vi "View AI param short.vi"(7 "ActivateAIView":bool, 9 "AIP":T1, 10 "AI_State":T3[](array[typedef]), 11 "AITable":dbl[](array[numeric]) format="%#.0f") -> (2 "Reread out":bool, 3 "This VI":refnum<vi>)   [LabVIEW 2019, in "Inputs.lvlib"]
uses:
  Inputs.lvlib
  Ctl/Parameter State.ctl
  Ctl/AI.ctl
  Ctl/AI short.ctl
  Database/Progress.vi
  Database/PostgreSQL.lvlib
  Logik/Logik.lvlib
panel:
  out "AI progress":i32(slide) scale=0.0..100.0
  in  "Reread":bool
  in  "n_elem":i32(c297)
  out "units":string[](array[string])
  out "AI_9":dbl format="%#.1f"
  out "AI_10":dbl format="%#.1f"
  out "AI_5":dbl format="%#.1f"
  out "AI_6":dbl format="%#.1f"
  out "AI_7":dbl format="%#.1f"
  out "AI_8":dbl format="%#.1f"
  out "AI_3":dbl format="%#.1f"
  out "AI_4":dbl format="%#.1f"
  out "AI_2":dbl format="%#.1f"
  out "AI_1":dbl format="%#.1f"
  out "n param":i32
  out "Names":string[](array[string])
  out "fcode":string[](array[string])
  out "Parameters table":dbl[][](array[numeric])=[[1.0, 0.0, 1000.0, 2.0, 0.0, 0.0, 2.0, 20.0, 100.0, nan, 250.0, 250.0, 2.0, 1.0, 10.0, 0.0, 65535.0, 0.0, 250.0, 1.0, 4.0], [1.0, 0.0, 1000.0, 2.0, 0.0, 0.0, 2.0, 20.0, 150.0, nan, 250.0, 250.0, 2.0, 1.0, 11.0, 0.0, 65535.0, 0.0, 250.0, 0.0, 4.0], [1.0, 0.0, 1000.0, 2.0, 0.0, 0.0, 2.0, 3.0, 7.0, 8.0, 10.0, 10.0, 2.0, 0.1, 1.0, 0.0, 65535.0, 0.0, 10.0, 0.0, 2.0], [1.0, 0.0, 1000.0, 2.0, 0.0, 0.0, 1.5, 2.5, 6.0, 7.0, 10.0, 10.0, 2.0, 0.1, 2.0, 0.0, 65535.0, 0.0, 10.0, 0.0, 3.0], [1.0, 0.0, 1000.0, 2.0, 0.0, 0.0, 2.0, 2.5, 6.0, 7.0, 10.0, 10.0, 2.0, 0.1, 3.0, 0.0, 65535.0, 0.0, 10.0, 1.0, 2.0], [1.0, 0.0, 1000.0, 2.0, 0.0, 0.0, 1.5, 2.0, 4.0, 5.0, 10.0, 10.0, 2.0, 0.1, 4.0, 0.0, 65535.0, 0.0, 10.0, 1.0, 3.0], [1.0, 0.0, 1000.0, 2.0, 0.0, 0.0, 3.0, 4.0, 8.0, 9.0, 10.0, 10.0, 2.0, 0.1, 5.0, 0.0, 65535.0, 0.0, 100.0, 1.0, 7.0], [1.0, 0.0, 1000.0, 2.0, 0.0, 0.0, 4.0, 8.0, nan, nan, 100.0, 100.0, 2.0, 1.0, 6.0, 0.0, 65535.0, 0.0, 100.0, 0.0, 0.0], [1.0, 0.0, 1000.0, 2.0, 0.0, 0.0, nan, nan, nan, nan, 100.0, 100.0, 2.0, 1.0, 7.0, 0.0, 65535.0, 0.0, 100.0, 0.0, 1.0], [1.0, 0.0, 1000.0, 2.0, 0.0, 0.0, nan, nan, nan, nan, 100.0, 100.0, 2.0, 1.0, 8.0, 0.0, 65535.0, 0.0, 100.0, 1.0, 0.0], [1.0, 0.0, 1000.0, 2.0, 0.0, 0.0, 10.0, 15.0, 45.0, 50.0, 100.0, 100.0, 2.0, 1.0, 9.0, 0.0, 65535.0, 0.0, 100.0, 1.0, 1.0]]
  # "time_const"
  # "0%"
  # "LL"
  # "L"
  # "OK"
  # "H"
  # "HH"
  # "100 %"
  # "d"
  # "Analog parameters"
  # "Description of analog parameters"
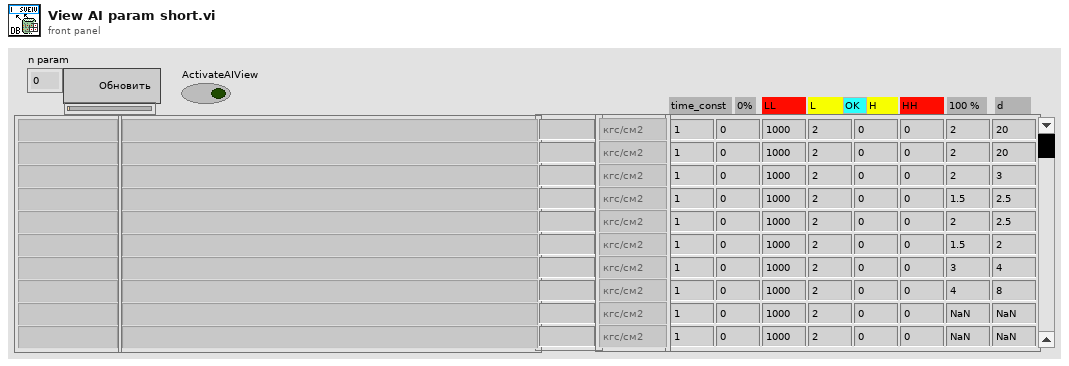
[diagram p1: front panel]
types:
  T1 = typedef "Inputs.lvlib/AI.ctl" = cluster{"AI_defs":T2, "modified":refnum<data-value>, "AIP":refnum<data-value>, "AINames":refnum<data-value>}
  T2 = typedef "Inputs.lvlib/AI short.ctl" = cluster{"AI":dbl[], "AIState":T3[], "AIALRState":errorcluster[]}
  T3 = typedef "Inputs.lvlib/Parameter State.ctl" = cluster{"code":i32, "visible":bool, "color":u32, "source":string}
  T4 = enum32{"Invalid", "Standard", "Closed", "Hidden", "Minimized", "Maximized"}
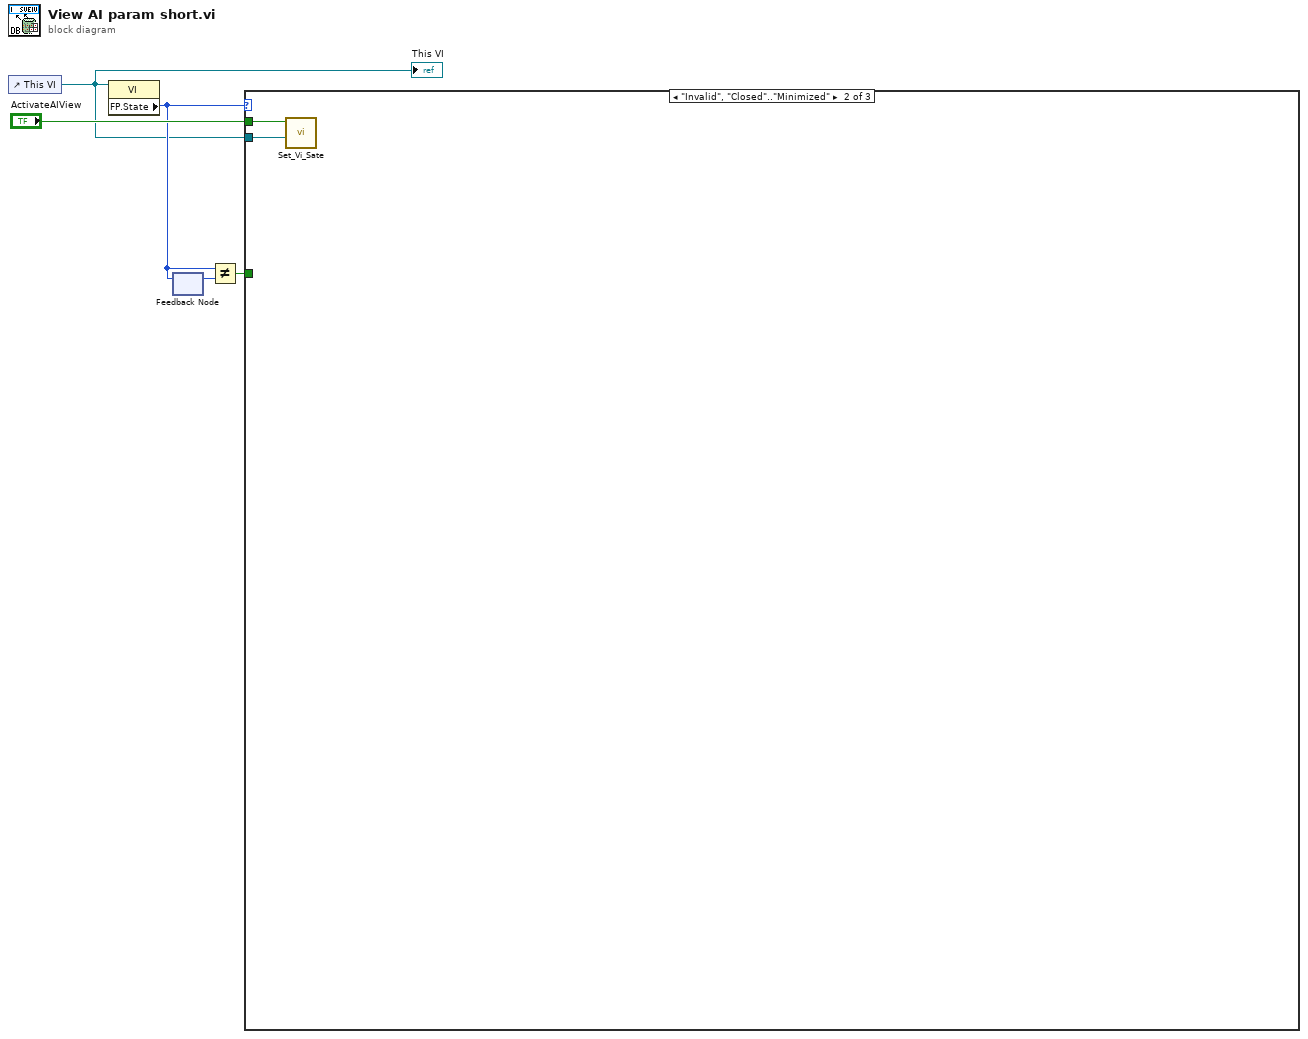
[diagram p0: block diagram]
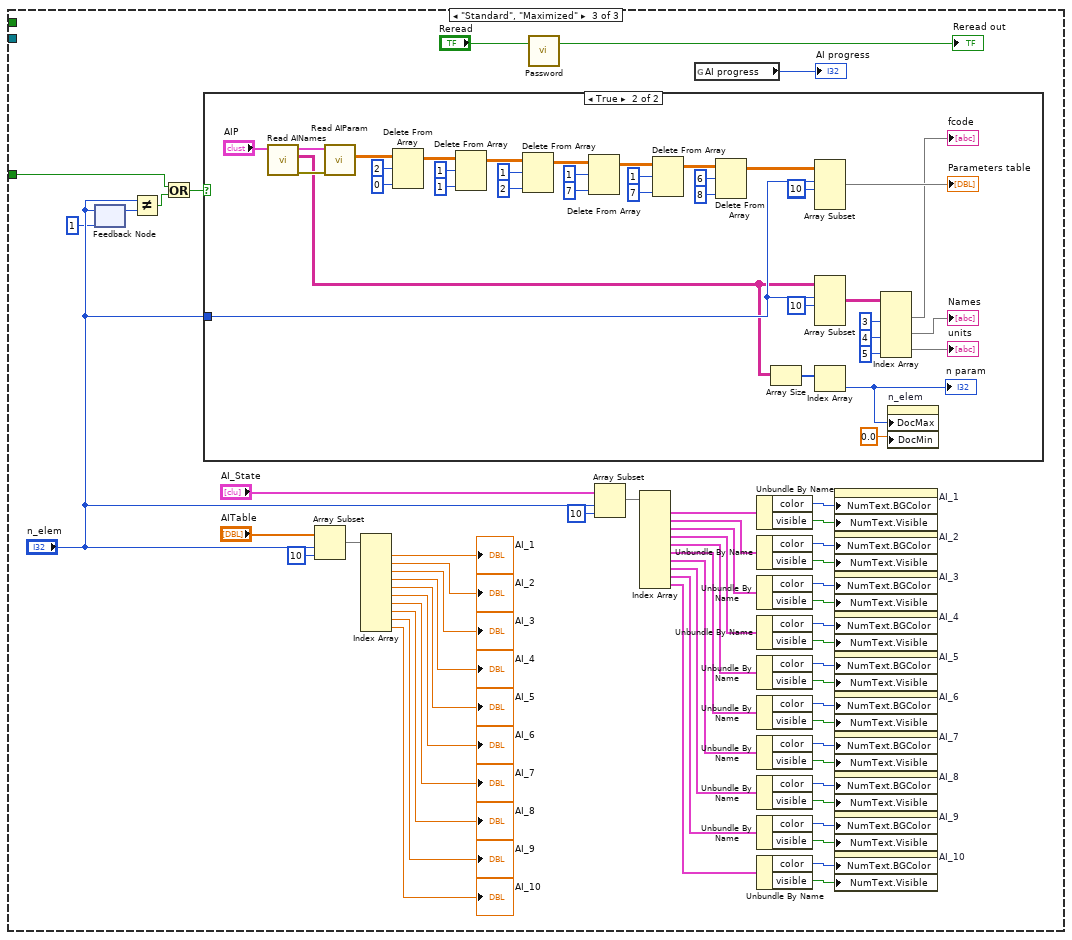
[diagram p3: hidden frame]
diagram:
  n1 = control-ref of="This VI"() -> (w1:refnum<vi>)
  "This VI" <- w1
  n2 = property class="VI"(reference=w1) -> ("FP.State"=w3:T4)  [unwired: 1 in, 2 out]
  n3 = feedback #1() -> (w4:T4)  [unwired: 1 in]
  n4 = feedback-in #1(w3) -> ()
  n5 = Not Equal?(x=w3, y=w4) -> (x != y?=w2:bool)
  n6 = case shown="\"Invalid\", \"Closed\"..\"Minimized\"" w3 {
    tunnel: "ActivateAIView" -> [_ w6 _]
    tunnel: w1 -> [_ w7 _]
    tunnel: w2 -> [_ _ w9]
    frame Default {
    }
    frame "Invalid", "Closed".."Minimized" {
      n7 = call "Set_Vi_Sate.vi"("VI"=w7, "Activate (F)"=w6) -> ()  [unwired: 9 in, 1 out]
    }
    frame "Standard", "Maximized" {
      n8 = feedback #2(1 ("n_elem")) -> (w14:i32)
      n9 = feedback-in #2("n_elem") -> ()
      n10 = Not Equal?(x="n_elem", y=w14) -> (x != y?=w11:bool)
      n11 = Or(x=w9, y=w11) -> (x .or. y?=w10:bool)
      n12 = case shown="True" w10 {
        tunnel: "n_elem" -> [_ w94]
        frame False {
        }
        frame True {
          (unwired) 10 ("length")
          n13 = call "Read AINames.vi"("AI in"="AIP") -> ("error out"=w66:errorcluster, "AINames"=w63:string[][], "AI out"=w64:T1)  [unwired: 8 in]
          n14 = call "Read AIParam.vi"("error in (no error)"=w66, "AI in"=w64) -> ("AIParam"=w67:dbl[][])  [unwired: 7 in, 2 out]
          n15 = Delete From Array(array=w67, length=2, index (col)=0 ("disabled index (col)")) -> (array with subset deleted=w73:dbl[][])  [unwired: 1 in, 1 out]
          n16 = Delete From Array(array=w73, length=1, index (col)=1 ("disabled index (col)")) -> (array with subset deleted=w80:dbl[][])  [unwired: 1 in, 1 out]
          n17 = Delete From Array(array=w80, length=1, index (col)=2 ("disabled index (col)")) -> (array with subset deleted=w81:dbl[][])  [unwired: 1 in, 1 out]
          n18 = Delete From Array(array=w81, length=1, index (col)=7 ("disabled index (col)")) -> (array with subset deleted=w83:dbl[][])  [unwired: 1 in, 1 out]
          n19 = Delete From Array(array=w83, length=1, index (col)=7 ("disabled index (col)")) -> (array with subset deleted=w84:dbl[][])  [unwired: 1 in, 1 out]
          n20 = Delete From Array(array=w84, length=6, index (col)=8 ("disabled index (col)")) -> (array with subset deleted=w92:dbl[][])  [unwired: 1 in, 1 out]
          n21 = Array Size(array=w63) -> (size(s)=w86:i32[])
          n22 = Array Subset(array=w92, index (row)=w94, length (row)=10 ("length")) -> (→"Parameters table":dbl[][])  [unwired: 2 in]
          n23 = Array Subset(array=w63, index (row)=w94, length (row)=10 ("length")) -> (w99:string[][])  [unwired: 2 in]
          n24 = Index Array(array=w86) -> (element=w85:i32)  [unwired: 1 in]
          "n param" <- w85
          n25 = Index Array(array=w99, index (col) #1=3 ("disabled index (col)"), index (col) #2=4 ("disabled index (col)"), index (col) #3=5 ("index (col)")) -> (element #1=→"fcode":string[], element #2=→"Names":string[], element #3=→"units":string[])  [unwired: 3 in]
          n26 = property on="n_elem" class="Scroll (strict)"("DocMax"=w85, "DocMin"=0.0 ("Data Entry Limits:Minimum")) -> ()  [unwired: 2 in, 2 out]
        }
      }
      n27 = Array Subset(array="AITable", index="n_elem", length=10) -> (w51:dbl[])
      n28 = Index Array(array=w51) -> (element #1=→"AI_1":dbl, element #2=→"AI_2":dbl, element #3=→"AI_3":dbl, element #4=→"AI_4":dbl, element #5=→"AI_5":dbl, element #6=→"AI_6":dbl, element #7=→"AI_7":dbl, element #8=→"AI_8":dbl, element #9=→"AI_9":dbl, element #10=→"AI_10":dbl)  [unwired: 10 in]
      n29 = call "Password.vi"("ActivatePASSWView"="Reread") -> ("enable"=→"Reread out":bool)  [unwired: 1 in, 1 out]
      n30 = Array Subset(array="AI_State", index="n_elem", length=10) -> (w22:T3[])
      n31 = Index Array(array=w22) -> (element #1=w23:T3, element #2=w24:T3, element #3=w25:T3, element #4=w44:T3, element #5=w45:T3, element #6=w46:T3, element #7=w47:T3, element #8=w48:T3, element #9=w49:T3, element #10=w50:T3)  [unwired: 10 in]
      n32 = global read "Progress.vi" "AI progress"() -> (→"AI progress":i32)
      n33 = Unbundle By Name(w23) -> ("color"=w17:u32, "visible"=w18:bool)
      n34 = Unbundle By Name(w24) -> ("color"=w26:u32, "visible"=w27:bool)
      n35 = Unbundle By Name(w25) -> ("color"=w28:u32, "visible"=w29:bool)
      n36 = Unbundle By Name(w44) -> ("color"=w30:u32, "visible"=w31:bool)
      n37 = Unbundle By Name(w45) -> ("color"=w32:u32, "visible"=w33:bool)
      n38 = Unbundle By Name(w46) -> ("color"=w34:u32, "visible"=w35:bool)
      n39 = Unbundle By Name(w47) -> ("color"=w36:u32, "visible"=w37:bool)
      n40 = Unbundle By Name(w48) -> ("color"=w38:u32, "visible"=w39:bool)
      n41 = Unbundle By Name(w49) -> ("color"=w40:u32, "visible"=w41:bool)
      n42 = Unbundle By Name(w50) -> ("color"=w42:u32, "visible"=w43:bool)
      n43 = property on="AI_1" class="DigNum (strict)"("NumText.BGColor"=w17, "NumText.Visible"=w18) -> ()  [unwired: 2 in, 2 out]
      n44 = property on="AI_2" class="DigNum (strict)"("NumText.BGColor"=w26, "NumText.Visible"=w27) -> ()  [unwired: 2 in, 2 out]
      n45 = property on="AI_3" class="DigNum (strict)"("NumText.BGColor"=w28, "NumText.Visible"=w29) -> ()  [unwired: 2 in, 2 out]
      n46 = property on="AI_4" class="DigNum (strict)"("NumText.BGColor"=w30, "NumText.Visible"=w31) -> ()  [unwired: 2 in, 2 out]
      n47 = property on="AI_5" class="DigNum (strict)"("NumText.BGColor"=w32, "NumText.Visible"=w33) -> ()  [unwired: 2 in, 2 out]
      n48 = property on="AI_6" class="DigNum (strict)"("NumText.BGColor"=w34, "NumText.Visible"=w35) -> ()  [unwired: 2 in, 2 out]
      n49 = property on="AI_7" class="DigNum (strict)"("NumText.BGColor"=w36, "NumText.Visible"=w37) -> ()  [unwired: 2 in, 2 out]
      n50 = property on="AI_8" class="DigNum (strict)"("NumText.BGColor"=w38, "NumText.Visible"=w39) -> ()  [unwired: 2 in, 2 out]
      n51 = property on="AI_9" class="DigNum (strict)"("NumText.BGColor"=w40, "NumText.Visible"=w41) -> ()  [unwired: 2 in, 2 out]
      n52 = property on="AI_10" class="DigNum (strict)"("NumText.BGColor"=w42, "NumText.Visible"=w43) -> ()  [unwired: 2 in, 2 out]
    }
  }
